vi "Command-Line Get Boolean Key.vi"(4 "boolean key":string) -> (0 "key found?":bool, 2 "boolean value":bool)   [LabVIEW 2015]
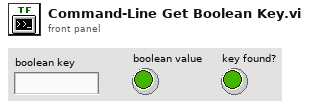
[diagram p1: front panel]
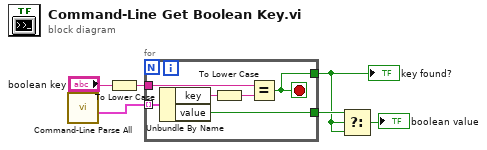
[diagram p0: block diagram]
diagram:
  n1 = call "Command-Line Parse All.vi"() -> ("boolean keys"=w3:cluster{"key":string, "value":bool}[])  [unwired: 6 in, 5 out]
  n2 = To Lower Case(string="boolean key") -> (all lower case string=w6:string)
  n3 = for {
    tunnel: w3 -> [w12] mode=indexing
    tunnel: w6 -> [w9]
    tunnel: [w8] -> w1
    tunnel: [w7] -> w4
    stop <- w8 stop-if-true
    n4 = Unbundle By Name(w12) -> ("key"=w11:string, "value"=w7:bool)
    n5 = To Lower Case(string=w11) -> (all lower case string=w10:string)
    n6 = Equal?(x=w9, y=w10) -> (x = y?=w8:bool)
  }
  "key found?" <- w1
  n7 = Select(t=w4, s=w1, f=w1) -> (s? t:f=→"boolean value":bool)
